vi "select_desired_frequency.vi"(9 "desired frequency":dbl format="%#_13g", 10 "FFT phase":cluster{"f0":dbl, "df":dbl, "phase":dbl[]}, 11 "FFT magnitude":cluster{"f0":dbl, "df":dbl, "magnitude":dbl[]}) -> (1 "actual frequency selected":dbl, 2 "output phase":dbl, 3 "output magnitude":dbl)   [LabVIEW 2021]
panel:
  out "index":dbl
  # "Inputs:"
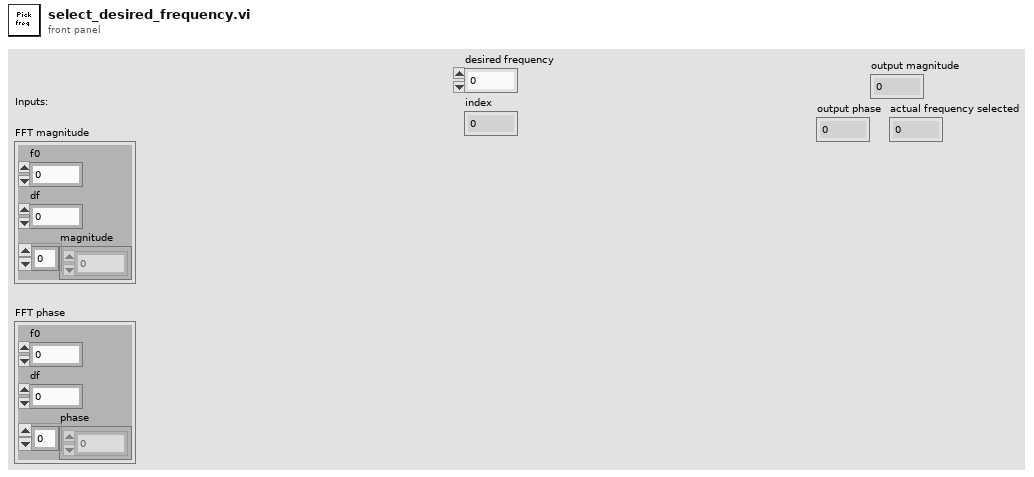
[diagram p1: front panel]
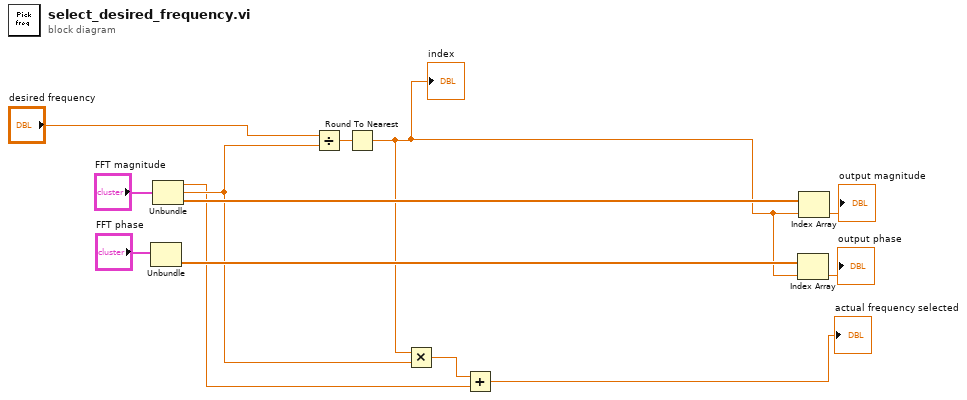
[diagram p0: block diagram]
diagram:
  n1 = Unbundle("FFT phase") -> ("phase"=w9:dbl[])  [unwired: 2 out]
  n2 = Unbundle("FFT magnitude") -> ("f0"=w2:dbl, "df"=w4:dbl, "magnitude"=w10:dbl[])
  n3 = Divide(x="desired frequency", y=w4) -> (x/y=w11:dbl)
  n4 = Round To Nearest(number=w11) -> (nearest integer value=w5:dbl)
  "index" <- w5
  n5 = Multiply(x=w5, y=w4) -> (x*y=w3:dbl)
  n6 = Add(x=w3, y=w2) -> (x+y=→"actual frequency selected":dbl)
  n7 = Index Array(array=w9, index=w5) -> (element=→"output phase":dbl)
  n8 = Index Array(array=w10, index=w5) -> (element=→"output magnitude":dbl)
